vi "add highlighting info.vi"(0 "data":cluster{"Y":i32, "X":i32, "Text":string}[](array[cluster]), 5 "Cursor Position":cluster{i32, i32}, 9 "Reset Selection":bool, 11 "error out":errorcluster) -> (1 "Updated Cursor Position":cluster{i32, i32}, 2 "Selection Position":cluster{i32, i32}, 3 "selected string":string, 4 "Array":T1(array[cluster]), 8 "Array 2":string[](array[string]), 15 "error IO":errorcluster)   [LabVIEW 2018]
uses:
  CAEN globals.vi
  <userlib>/_OpenG.lib/array/array.llb/Search 1D Array (Boolean)__ogtk.vi
  <userlib>/_OpenG.lib/array/array.llb/Search 1D Array (String)__ogtk.vi
  <userlib>/_OpenG.lib/array/array.llb/Index 1D Array Elements (I32)__ogtk.vi
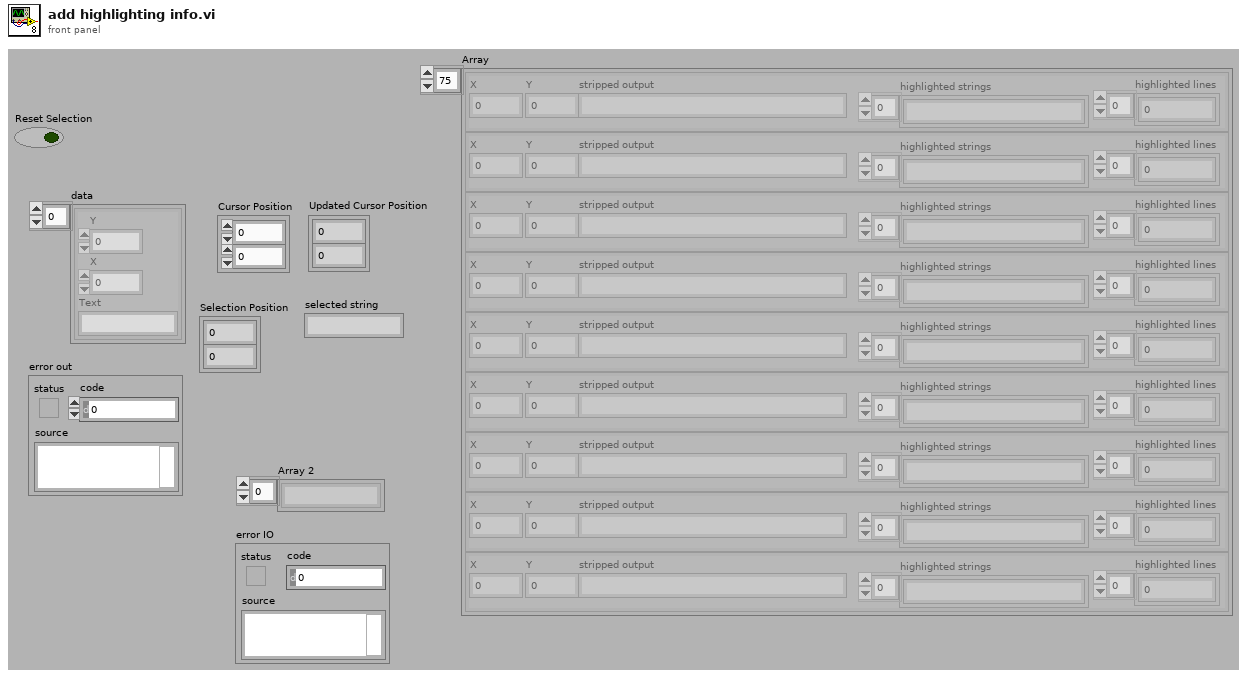
[diagram p1: front panel]
types:
  T1 = cluster{"Y":i32, "X":i32, "stripped output":string, "highlighted strings":string[], "highlighted lines":i32[]}[]
  T2 = cluster{"Y":i32, "X":i32, "stripped output":string, "highlighted strings":string[], "highlighted lines":i32[]}
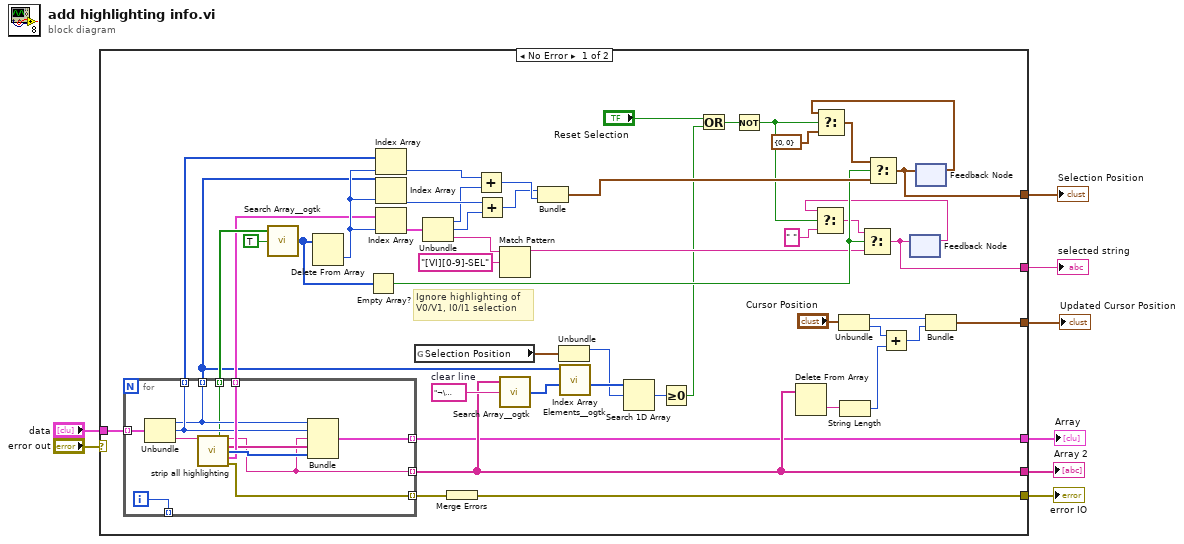
[diagram p0: block diagram]
diagram:
  n1 = case shown="No Error" "error out" {
    selector: "error out" -> [_ w70]
    tunnel: [w18 w70] -> w5
    tunnel: [w9 _] -> w8
    tunnel: [w10 _] -> w6
    tunnel: "data" -> [w56 _]
    tunnel: [w31 _] -> w3
    tunnel: [w41 _] -> w2
    tunnel: [w13 _] -> w1
    frame No Error {
      w29 = "¬\u001b[K"  # clear line
      # "Ignore highlighting of\nV0/V1, I0/I1 selection"
      n2 = for {
        tunnel: [w59] -> w57 mode=indexing
        tunnel: [w69] -> w9 mode=indexing
        tunnel: [w58] -> w10 mode=indexing
        tunnel: w56 -> [w68] mode=indexing
        tunnel: [w66] -> w33 mode=indexing
        tunnel: [w63] -> w27 mode=indexing
        tunnel: [w62] -> w54 mode=indexing
        tunnel: [w64] -> w32 mode=indexing
        tunnel: [w61] -> _ mode=indexing
        i -> [w61]
        n3 = Unbundle(w68) -> ("Y"=w63:i32, "X"=w64:i32, "Text"=w65:string)
        n4 = call "strip all highlighting.vi"("input string"=w65) -> ("Selection"=w62:bool, "stripped output"=w58:string, "highlighted strings"=w60:string[], "highlighted lines"=w67:i32[], "Selection cluster"=w66:cluster{i32, i32, "selected string":string}, "error out"=w59:errorcluster)  [unwired: 9 in]
        n5 = Bundle("Y"=w63, "X"=w64, "stripped output"=w58, "highlighted strings"=w60, "highlighted lines"=w67) -> (w69:T2)  [unwired: 1 in]
      }
      n6 = call-poly <userlib>:"Search Array__ogtk.vi"("Array"=w54, "Element Data"=TRUE ("element")) -> ("Indices of Elements"=w40:i32[])  [unwired: 7 in]
      n7 = Delete From Array(array=w40) -> (deleted portion=w45:i32)  [unwired: 2 in, 1 out]
      n8 = Empty Array?(array=w40) -> (empty?=w43:bool)
      n9 = Index Array(array=w32, index=w45) -> (element=w52:i32)
      n10 = Index Array(array=w27, index=w45) -> (element=w51:i32)
      n11 = Index Array(array=w33, index=w45) -> (element=w53:cluster{i32, i32, "selected string":string})
      n12 = global read "CAEN globals.vi" "Selection Position"() -> (w19:cluster{i32, i32})
      n13 = Unbundle(w53) -> (w49:i32, w50:i32, "selected string"=w48:string)
      n14 = Merge Errors(w57) -> (w18:errorcluster)
      n15 = Add(x=w52, y=w49) -> (x+y=w46:i32)
      n16 = Add(x=w51, y=w50) -> (x+y=w30:i32)
      n17 = Match Pattern(string=w48, regular expression="[VI][0-9]-SEL") -> (before substring=w42:string)  [unwired: 1 in, 3 out]
      n18 = call-poly <userlib>:"Search Array__ogtk.vi"("Array"=w10, "Element Data"=w29) -> ("Indices of Elements"=w28:i32[])  [unwired: 7 in]
      n19 = Bundle(w30, w46) -> (w44:cluster{i32, i32})  [unwired: 1 in]
      n20 = Unbundle(w19) -> (w25:i32)  [unwired: 1 out]
      n21 = call-poly <userlib>:"Index Array Elements__ogtk.vi"("indices"=w28, "array"=w27) -> ("elements"=w26:i32[])  [unwired: 9 in]
      n22 = Search 1D Array(1D array=w26, element=w25) -> (index of element=w24:i32)  [unwired: 1 in]
      n23 = Greater Or Equal To 0?(x=w24) -> (x >= 0?=w23:bool)
      n24 = Or(x="Reset Selection", y=w23) -> (x .or. y?=w21:bool)
      n25 = Not(x=w21) -> (.not. x?=w20:bool)
      n26 = Delete From Array(array=w10) -> (deleted portion=w16:string)  [unwired: 2 in, 1 out]
      n27 = Unbundle("Cursor Position") -> (w17:i32, w15:i32)
      n28 = String Length(string=w16) -> (length=w12:i32)
      n29 = Add(x=w15, y=w12) -> (x+y=w14:i32)
      n30 = feedback #1() -> (w36:string)  [unwired: 1 in]
      n31 = Select(t=w36, s=w20, f=" ") -> (s? t:f=w35:string)
      n32 = Select(t=w35, s=w43, f=w42) -> (s? t:f=w41:string)
      n33 = feedback-in #1(w41) -> ()
      n34 = feedback #2() -> (w38:cluster{i32, i32})  [unwired: 1 in]
      n35 = Select(t=w38, s=w20, f=cluster{i32, i32} {0, 0}) -> (s? t:f=w39:cluster{i32, i32})
      n36 = Select(t=w39, s=w43, f=w44) -> (s? t:f=w31:cluster{i32, i32})
      n37 = feedback-in #2(w31) -> ()
      n38 = Bundle(w17, w14) -> (w13:cluster{i32, i32})  [unwired: 1 in]
    }
    frame Error {
    }
  }
  "Array" <- w8
  "Array 2" <- w6
  "error IO" <- w5
  "Selection Position" <- w3
  "selected string" <- w2
  "Updated Cursor Position" <- w1
